vi "Rms_calculation.vi"(1 "Vabc":T1) -> (0 "Three phase RMS":fxp<+,27,5>)   [LabVIEW 2015]
uses:
  <vilib>/rvi/FXPMathLib/FxpSqrt/subVIs/nifxpmath_Sqrt_SimConfig.ctl
  <vilib>/fxp/LVFixedPointOverflowPolicyTypeDef.ctl
  <vilib>/rvi/Emulation/niFpgaGetClockAttributes.vi
  <vilib>/rvi/Emulation/niFpgaSctlEmulationGetInTimedLoop.vi
  <vilib>/rvi/Emulation/niFpgaEmulationReportErrorSimple.vi
  <vilib>/rvi/FXPMathLib/FxpSqrt/simVIs/DllSqrtTemp_sub.vi
  <vilib>/rvi/Emulation/niFpgaCriticalErrorInLSC.vi
  <vilib>/rvi/FXPMathLib/FxpAdd/XNode/nifxpmath_Add.xnode
  <vilib>/rvi/FXPMathLib/FxpMul/XNode/nifxpmath_Multiplier.xnode
  <vilib>/rvi/FXPMathLib/FxpSqrt/XNode/nifxpmath_Sqrt.xnode
  <vilib>/rvi/FXPMathLib/sim/FxpSim.dll
types:
  T1 = cluster{"A":fxp<+/-,18,4>, "B":fxp<+/-,18,4>, "C":fxp<+/-,18,4>}
  T2 = cluster{"A":fxp<+,35,7>, "B":fxp<+,35,7>, "C":fxp<+,35,7>}
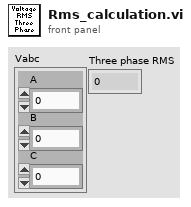
[diagram p1: front panel]
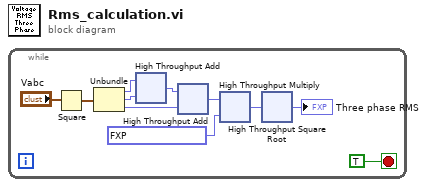
[diagram p0: block diagram]
diagram:
  n1 = while {
    stop <- TRUE stop-if-true
    n2 = Square(x="Vabc") -> (x^2=w10:T2)
    n3 = Unbundle(w10) -> ("A"=w9:fxp<+,35,7>, "B"=w8:fxp<+,35,7>, "C"=w6:fxp<+,35,7>)
    n4 = xnode "High Throughput Add"("x"=w9, "y"=w8) -> ("x+y"=w7:fxp<+,36,8>)
    n5 = xnode "High Throughput Add"("x"=w7, "y"=w6) -> ("x+y"=w5:fxp<+,37,9>)
    n6 = xnode "High Throughput Multiply"("x"=w5, "y"=fxp<+,16,1> 0.33331298828125) -> ("x*y"=w3:fxp<+,53,10>)
    n7 = xnode "High Throughput Square Root"("x"=w3) -> ("sqrt(x)"=→"Three phase RMS":fxp<+,27,5>)
  }
